vi "Read Section Cluster__lvcfg.vi"(7 "section (optional)":string, 8 "error in (no error)":errorcluster, 10 "Section Formatted Cluster Type":variant, 11 "Config in":T1) -> (0 "error out":errorcluster, 1 "all found?":bool, 2 "Section Formatted Cluster":variant, 3 "Config out":T1, 4 "any found?":bool)   [LabVIEW 2017, in "LabVIEW Config(Variant).lvlib"]
doc: "Reads key-value pairs from a section of the configuration data identified by refnum, and returns them as a cluster of items. If \"key\" input is not specified, the name of the cluster within the \"Section Formatted Cluster type\" input is used as the key. Only the items within the \"Section Formatted Cluster Type\" input cluster are read from the configuration data and returned in the output cluster. The \"found?\" output will be TRUE only if all elements (recursively) are found.\n\nFor example an section cluster named \"MyCluster1\" contains two elements named \"MyNumeric\" and \"MyBoolean\". This would correspond to an INI read of the following data:\n\n[MyCluster1]\nMyNumeric=1.024\nMyBoolean=TRUE\n\nNote: Special characters in section and key names will be escape-coded. These include the following: \\00-\\1F (non-printable chars); \"[\", \"]\", and \"=\" (INI syntax elements); \\FE (\"þ\") and \\FF (\"ÿ\") (legacy bracket encoding); Additionally, the escape character, \"\\\", will be escaped as \"\\\\\"."
uses:
  LabVIEW Config(Variant).lvlib
  <userlib>/_NEVSTOP/Communicable State Machine(CSM)/addons/INI-Static-Variable-Support/LabVIEW-Config/Config.ctl
  <userlib>/_NEVSTOP/Communicable State Machine(CSM)/Communicable State Machine.lvlib
  <userlib>/_NEVSTOP/Communicable State Machine(CSM)/addons/INI-Static-Variable-Support/LabVIEW-Config/LabVIEW-Config.lvlib
panel:
  # "Read Section Cluster.vi\n\nReads an INI section cluster (variant) from INI file.\n\nPlease visit http://www.OpenG.org to learn about the\nOpen Source LabVIEW software movement.\n\nNOTICE -- YOU MUST LEAVE THIS NOTICE IN PLACE.  PER THE TERMS OF THE LICENSE BELOW, YOU MAY SUBLICENSE THIS SOFTWARE \nIN ANY WAY THAT DOES NOT CONFLICT WITH THIS LICENSE.\n\n### BSD License (http://www.opensource.org/licenses/bsd-license.php) Begin ###\n \nCopyright (c) 2002-2006, Jim Kring <jim@jimkring.com>\n\nAll rights reserved.\n\nRedistribution and use in source and binary forms, with or without modification, are permitted provided that the following conditions are met:\n\n    * Redistributions of source code must retain the above copyright notice, this list of conditions and the following disclaimer.\n    * Redistributions in binary form must reproduce the above copyright notice, this list of conditions and the following disclaimer in the \n       documentation and/or other materials provided with the distribution.\n    * Neither the name of SciWare, James Kring, Inc., nor the names of its contributors may be used to endorse or promote products derived \n       from this software without specific prior written permission.\n\nTHIS SOFTWARE IS PROVIDED BY THE COPYRIGHT HOLDERS AND CONTRIBUTORS \"AS IS\" AND ANY EXPRESS OR IMPLIED WARRANTIES, \nINCLUDING, BUT NOT LIMITED TO, THE IMPLIED WARRANTIES OF MERCHANTABILITY AND FITNESS FOR A PARTICULAR PURPOSE ARE \nDISCLAIMED. IN NO EVENT SHALL THE COPYRIGHT OWNER OR CONTRIBUTORS BE LIABLE FOR ANY DIRECT, INDIRECT, INCIDENTAL,\n SPECIAL, EXEMPLARY, OR CONSEQUENTIAL DAMAGES (INCLUDING, BUT NOT LIMITED TO, PROCUREMENT OF SUBSTITUTE GOODS OR \nSERVICES; LOSS OF USE, DATA, OR PROFITS; OR BUSINESS INTERRUPTION) HOWEVER CAUSED AND ON ANY THEORY OF LIABILITY, \nWHETHER IN CONTRACT, STRICT LIABILITY, OR TORT (INCLUDING NEGLIGENCE OR OTHERWISE) ARISING IN ANY WAY OUT OF THE USE \nOF THIS SOFTWARE, EVEN IF ADVISED OF THE POSSIBILITY OF SUCH DAMAGE.\n\n### BSD License End ###"
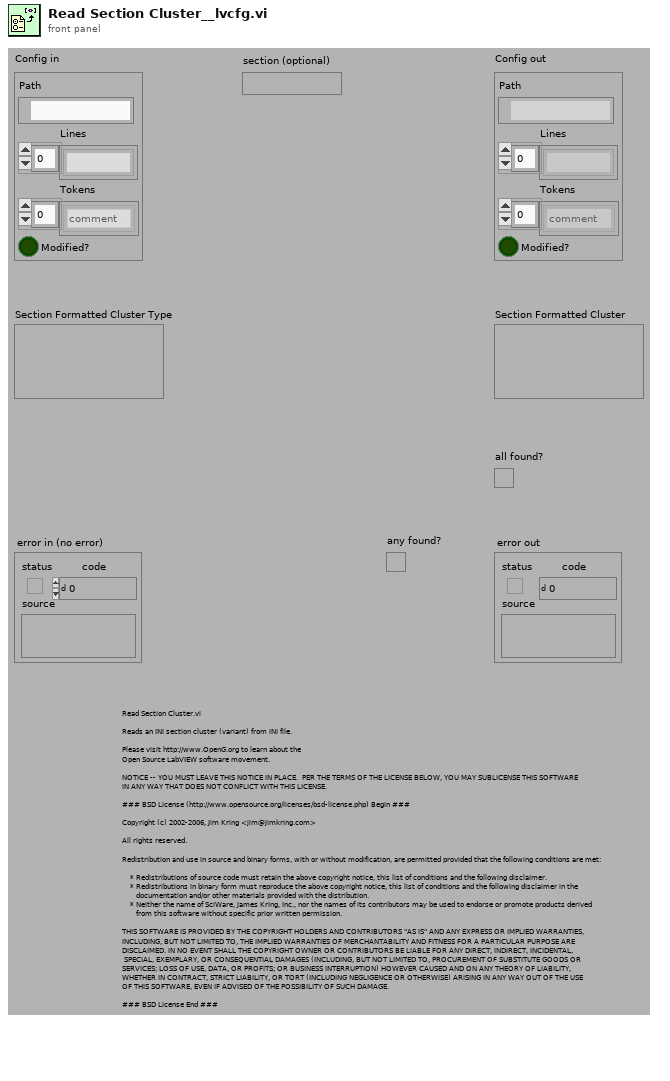
[diagram p1: front panel]
types:
  T1 = typedef "LabVIEW-Config.lvlib/Config.ctl" = cluster{"Path":path, "Lines":string[], "Tokens":enum8{"comment", "section", "key"}[], "Modified?":bool}
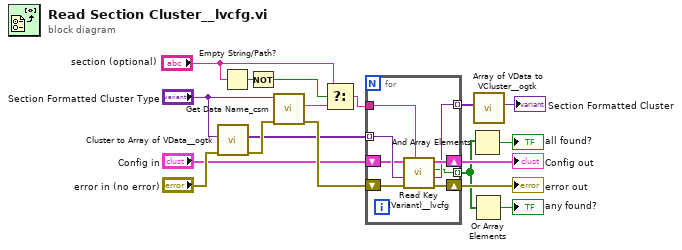
[diagram p0: block diagram]
diagram:
  n1 = call <userlib>:"Cluster to Array of VData__ogtk.vi"("error in (no error)"="error in (no error)", "Cluster"="Section Formatted Cluster Type") -> ("error out"=w16:errorcluster, "Array of VData"=w12:variant[])  [unwired: 8 in]
  n2 = Empty String/Path?(string/path="section (optional)") -> (empty?=w9:bool)
  n3 = Not(x=w9) -> (.not. x?=w7:bool)
  n4 = call <userlib>:"Get Data Name_csm.vi"("error in (no error)"=w16, "Data"="Section Formatted Cluster Type") -> ("error out"=w18:errorcluster, "Data Name"=w6:string)  [unwired: 7 in, 1 out]
  n5 = Select(t="section (optional)", s=w7, f=w6) -> (s? t:f=w5:string)
  n6 = for {
    tunnel: w12 -> [w26] mode=indexing
    shift-right: [w22] -> w14
    shift-left: "Config in" -> [w25]
    shift-right: [w23] -> w15
    shift-left: w18 -> [w24]
    tunnel: w5 -> [w21]
    tunnel: [w20] -> w11 mode=indexing
    tunnel: [w19] -> w2 mode=indexing
    n7 = call "Read Key (Variant)__lvcfg.vi"("section"=w21, "error in (no error)"=w24, "type"=w26, "Config in"=w25) -> ("error out"=w23:errorcluster, "key-value"=w20:variant, "found?"=w19:bool, "Config out"=w22:T1)  [unwired: 4 in]
  }
  "error out" <- w15
  "Config out" <- w14
  n8 = And Array Elements(Boolean array=w2) -> (logical AND=→"all found?":bool)
  n9 = Or Array Elements(Boolean array=w2) -> (logical OR=→"any found?":bool)
  n10 = call <userlib>:"Array of VData to VCluster__ogtk.vi"("Array"=w11) -> ("VCluster"=→"Section Formatted Cluster":variant)  [unwired: 9 in, 1 out]
